vi "Exit LabVIEW.vi"(8 "Error (Dependency Only)":errorcluster) -> ()   [LabVIEW 2020, in "Endigit.lvlib"]
doc: "This VI has no effect in the development environment. When in an executable, it closes the front panel and exits LabVIEW. This removes the need for the user to have to close an executable twice.\n\nAuthored by Robert C. Mortensen\nrobert@endigit.com\n\nCopyright (c) 2015, Endigit, Inc."
uses:
  Endigit.lvlib
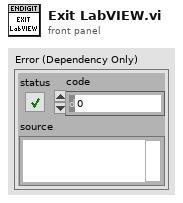
[diagram p1: front panel]
types:
  T1 = enum32{"invalid app kind", "Development System", "Run Time System", "Student Edition", "Embedded LabVIEW", "Evaluation", "Custom"}
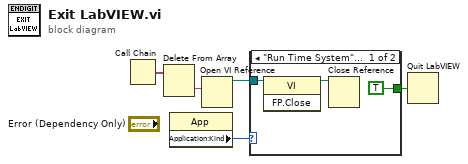
[diagram p0: block diagram]
diagram:
  n1 = Call Chain() -> (call chain=w3:string[])
  n2 = Delete From Array(array=w3) -> (deleted portion=w2:string)  [unwired: 2 in, 1 out]
  n3 = property class="App"() -> ("Application:Kind"=w5:T1)  [unwired: 2 in, 2 out]
  n4 = Open VI Reference(vi path=w2) -> (vi reference=w1:refnum<vi>)  [unwired: 5 in, 1 out]
  n5 = case shown="\"Run Time System\", \"Embedded LabVIEW\"" w5 {
    tunnel: w1 -> [w7 _]
    tunnel: [TRUE _] -> w4
    frame "Run Time System", "Embedded LabVIEW" {
      n6 = invoke class="VI" method="FP.Close"(reference=w7) -> (reference out=w8:refnum<vi>)  [unwired: 2 in, 2 out]
      n7 = Close Reference(reference=w8) -> ()  [unwired: 1 in, 1 out]
    }
    frame Default {
    }
  }
  n8 = Quit LabVIEW(quit? (T)=w4) -> ()
